vi "registerPublisher_old.vi"(1 "Parameters":T2) -> (2 "Error out":errorcluster, 3 "Reply":T1, 4 "Reply":string, 5 "registerPublisher":string)   [LabVIEW 2013]
uses:
  _ROSDefinition.vi
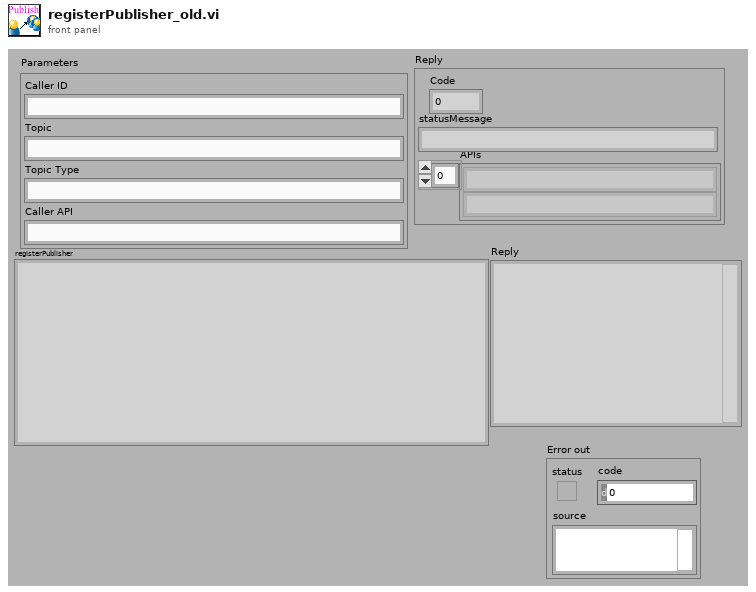
[diagram p1: front panel]
types:
  T1 = cluster{"Code":i8, "statusMessage":string, "APIs":string[]}
  T2 = cluster{"Caller ID":string, "Topic":string, "Topic Type":string, "Caller API":string}
  T3 = cluster{"Code":i8, "statusMessage":string, "APIs":string[]}[]
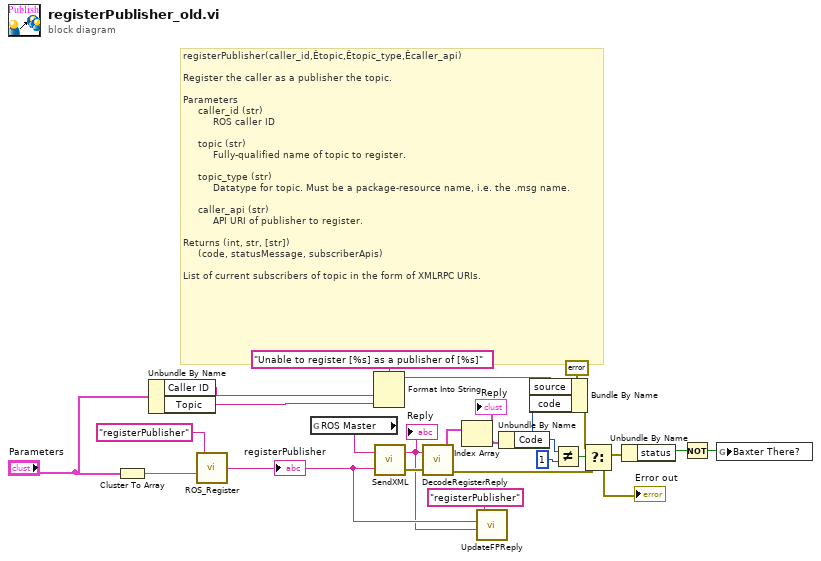
[diagram p0: block diagram]
diagram:
  # "registerPublisher(caller_id,Êtopic,Êtopic_type,Êcaller_api)\n\nRegister the caller as a publisher the topic. \n\nParameters \n     caller_id (str) \n          ROS caller ID\n\n     topic (str) \n          Fully-qualified name of topic to register.\n\n     topic_type (str) \n          Datatype for topic. Must be a package-resource name, i.e. the .msg name.\n\n     caller_api (str) \n          API URI of publisher to register.\n\nReturns (int, str, [str]) \n     (code, statusMessage, subscriberApis) \n\nList of current subscribers of topic in the form of XMLRPC URIs."
  n1 = Cluster To Array(cluster="Parameters") -> (array=w4:string[])
  n2 = Unbundle By Name("Parameters") -> ("Caller ID"=w21:string, "Topic"=w22:string)
  n3 = call "ROS_Register.vi"("Parameters"=w4, "Method Name"="registerPublisher") -> ("registerSubscriber"=w2:string)  [unwired: 1 in]
  "registerPublisher" <- w2
  n4 = global read "_ROSDefinition.vi" "ROS Master"() -> (w23:string)
  n5 = Format Into String(format string="Unable to register [%s] as a publisher of [%s]" ("source"), w21, w22) -> (resulting string=w11:string)  [unwired: 2 in, 1 out]
  n6 = call "SendXML.vi"("Send"=w2, "URI in"=w23) -> ("error out"=w17:errorcluster, "Reply"=w1:string)
  "Reply" <- w1
  n7 = call "DecodeRegisterReply.vi"("error in (no error)"=w17, "Response"=w1) -> ("error out"=w13:errorcluster, "Reply"=w16:T3)
  n8 = Index Array(array=w16) -> (element=w7:T1)  [unwired: 1 in]
  "Reply" <- w7
  n9 = call "UpdateFPReply.vi"("Reply"=w1, "Sent"=w2, "method"="registerPublisher" ("name (unnamed)")) -> ()  [unwired: 3 in]
  n10 = Unbundle By Name(w7) -> ("Code"=w10:i8)
  n11 = Bundle By Name(cluster=errorcluster {"status"=TRUE, "code"=0, "source"=" Error"} ("t"), "source"=w11, "code"=w10) -> (w9:errorcluster)
  n12 = Not Equal?(x=w10, y=i8 1) -> (x != y?=w14:bool)
  n13 = Select(t=w9, s=w14, f=w13) -> (s? t:f=w8:errorcluster)
  "Error out" <- w8
  n14 = Unbundle By Name(w8) -> ("status"=w18:bool)
  n15 = Not(x=w18) -> (.not. x?=w19:bool)
  n16 = global write "_ROSDefinition.vi" "Baxter There?"(w19) -> ()
